vi "get_event_description.vi"(6 "prepend string":string, 8 "error in (no error)":errorcluster, 9 "alternative message (used if control reference is empty)":string, 10 "event":T1, 11 "control reference in":refnum<vi>) -> (0 "error out":errorcluster, 2 "description":string, 3 "control reference out":refnum<vi>)   [LabVIEW 2010]
uses:
  <vilib>/event_ctls.llb/lveventtype.ctl
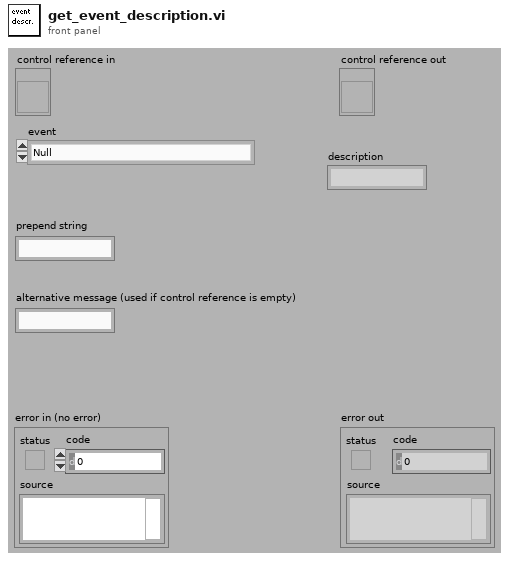
[diagram p1: front panel]
types:
  T1 = typedef "lveventtype.ctl" = enum32{"Null", "Timeout", "App Instance Close", "App Instance Close?", "Autoscale Range Change", "Cell Edit", "Cell Edit?", "Cursor Grab", "Cursor Grab?", "Cursor Move", "Cursor Release", "Data Change", "Direction Change", "Display State Change", "Drag Ended", "Drag Enter", "Drag Leave", "Drag Over", "Drag Source Update", "Drag Starting", "Drag Starting?", "Drop", "Exec State Change", "Key Down", "Key Down?", "Key Repeat", "Key Repeat?", "Key Up", "Listbox Double Click", "Menu Activation?", "Menu Selection (App)", "Menu Selection? (App)", "Menu Selection (User)", "Mouse Down", "Mouse Down?", "Mouse Enter", "Mouse Leave", "Mouse Move", "Mouse Up", "NI Security User Change (App)", "Pane Size", "Panel Close", "Panel Close?", "Panel Resize", "Plot Attribute Change", "Scale Range Change", "Shortcut Menu Activation?", "Shortcut Menu Selection (App)", "Shortcut Menu Selection? (App)", "Shortcut Menu Selection (User)", "Tree Double Click", "Tree Drag", "Tree Drag?", "Tree Drop", "Tree Drop?", "Tree Item Close", "Tree Item Close?", "Tree Item Open", "Tree Item Open?", "Value Change"}
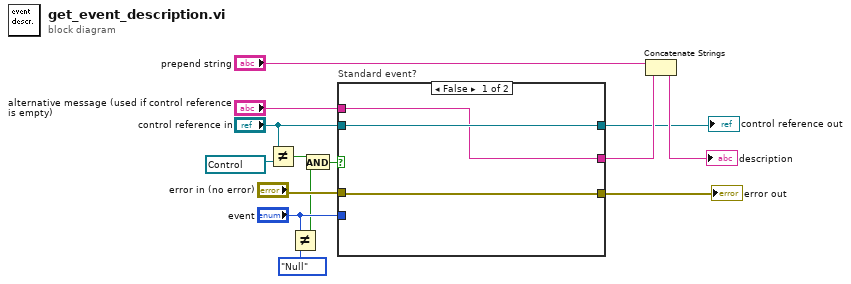
[diagram p0: block diagram]
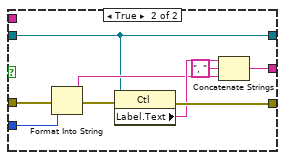
[diagram p2: hidden frame]
diagram:
  n1 = Not Equal?(x="control reference in", y=refnum<vi> refnum ("control reference in 2")) -> (x != y?=w4:bool)
  n2 = Not Equal?(x="event", y=lveventtype."Null" ("event 2")) -> (x != y?=w2:bool)
  n3 = And(x=w4, y=w2) -> (x .and. y?=w3:bool)
  n4 = case "Standard event?" shown="False" w3 {
    tunnel: "error in (no error)" -> [w15 w26]
    tunnel: [w15 w25] -> w13
    tunnel: "event" -> [_ w24]
    tunnel: [w16 w23] -> w11
    tunnel: "control reference in" -> [w17 w18]
    tunnel: [w17 w18] -> w9
    tunnel: "alternative message (used if control reference is empty)" -> [w16 _]
    frame False {
    }
    frame True {
      n5 = Format Into String(error in=w26, w24) -> (resulting string=w20:string, error out=w22:errorcluster)  [unwired: 2 in]
      n6 = property class="Ctl"(reference=w18, error in=w22) -> (error out=w25:errorcluster, "Label.Text"=w21:string)  [unwired: 1 out]
      n7 = Concatenate Strings(w21, ", " ("string"), w20) -> (w23:string)
    }
  }
  "error out" <- w13
  "control reference out" <- w9
  n8 = Concatenate Strings("prepend string", w11) -> (→"description":string)
